vi "Pockels Cal-Format cal table.vi"(10 "Calibration data (all objectives even if blank + inc. data header row)":string[][](array[string]), 11 "Pockels calibration voltage steps sequence (1st column)":string[](array[string])) -> (1 "Cancelled":bool, 3 "Formatted cal table (inc. header)":string[][](array[string]))   [LabVIEW 2013]
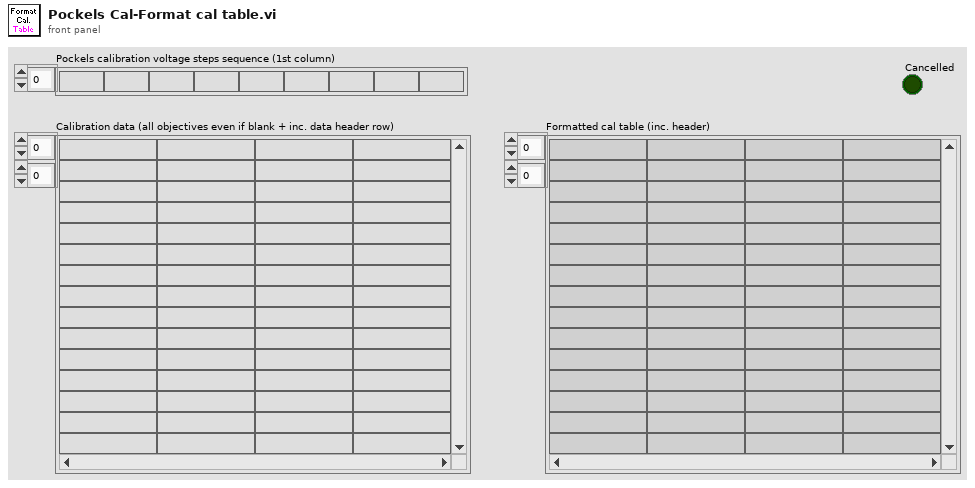
[diagram p1: front panel]
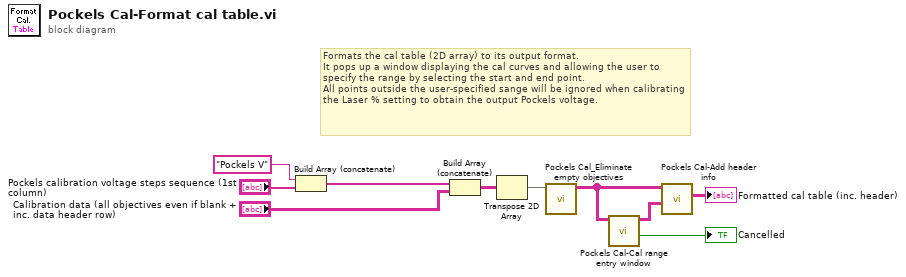
[diagram p0: block diagram]
diagram:
  # "Formats the cal table (2D array) to its output format.\nIt pops up a window displaying the cal curves and allowing the user to specify the range by selecting the start and end point.\nAll points outside the user-specified sange will be ignored when calibrating the Laser % setting to obtain the output Pockels voltage."
  n1 = Build Array (concatenate)("Pockels V", "Pockels calibration voltage steps sequence (1st column)") -> (w9:string[])
  n2 = Build Array (concatenate)(w9, "Calibration data (all objectives even if blank + inc. data header row)") -> (w7:string[][])
  n3 = Transpose 2D Array(2D array=w7) -> (transposed array=w3:string[][])
  n4 = call "Pockels Cal_Eliminate empty objectives.vi"("New cal section"=w3) -> ("New cal section"=w2:string[][])  [unwired: 10 in]
  n5 = call "Pockels Cal-Cal range entry window.vi"("Calibration data array (inc. data header row)"=w2) -> ("Cancelled"=→"Cancelled":bool, "Cal subset info array"=w4:string[][])  [unwired: 9 in]
  n6 = call "Pockels Cal-Add header info.vi"("Cal subset indexes info"=w4, "Calibration data array (inc. data header row)"=w2) -> ("Cal table (Final format)"=→"Formatted cal table (inc. header)":string[][])  [unwired: 9 in]
